vi "Write Cartesian Lines .vi"(5 "Cartesian Lines":bool, 9 "XYGraph in":refnum<class "XYGraph.lvclass">) -> (3 "XYGraph out":refnum<class "XYGraph.lvclass">)   [LabVIEW 2014, in "Raspberry Pi Compatible Compiler for LabVIEW.lvlib" / "XYGraph.lvclass"]
uses:
  XYGraph.lvclass
  XYGraph.lvclass/XYGraph.ctl
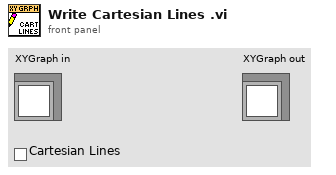
[diagram p1: front panel]
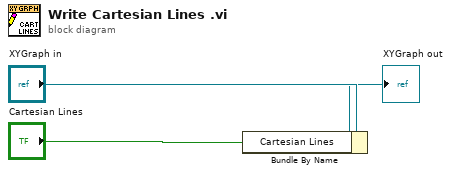
[diagram p0: block diagram]
diagram:
  n1 = Bundle By Name(cluster="XYGraph in", "Cartesian Lines"="Cartesian Lines") -> (→"XYGraph out":refnum<class "XYGraph.lvclass">)
